vi "Convert SS2 Data Info to String.vi"(5 "File Path":path, 6 "Step Duration":dbl[unit] format="%#.3g", 7 "Laser Period":dbl[unit], 8 "error in (no error)":errorcluster, 9 "size":i64, 10 "# Frames":u32, 11 "Swiss SPAD 2 File Information":T1 {"DAQ Parameters"."# Gate Positions" format="%0.0f"; "DAQ Parameters"."Gate Offset" format="%0.0f"; "DAQ Parameters"."Bitness" format="%0.0f"; "DAQ Parameters"."# Gate Set" format="%0.0f"; "FPGA Parameters"."gs_psincdec 3" format="%0.0f"; "FPGA Parameters"."gs_psincdec 2" format="%0.0f"; "FPGA Parameters"."gs_psincdec_1" format="%0.0f"; "FPGA Parameters"."gs_no_shift_adj_3" format="%0.0f"; "FPGA Parameters"."gs_no_shift_adj_2" format="%0.0f"; "FPGA Parameters"."gs_psincdec_0" format="%0.0f"}) -> (0 "Error Out":errorcluster, 3 "Data Description":string)   [LabVIEW 2021, in "SwissSPAD.lvlib"]
uses:
  SwissSPAD.lvlib
  SS2 File Information.ctl
  SS2 FPGA Parameters.ctl
  SS2 DAQ Parameters.ctl
  SS2 Data Information.ctl
  SwissSPAD 8-bit Frames Read.ctl
  Variant/Variant.lvlib
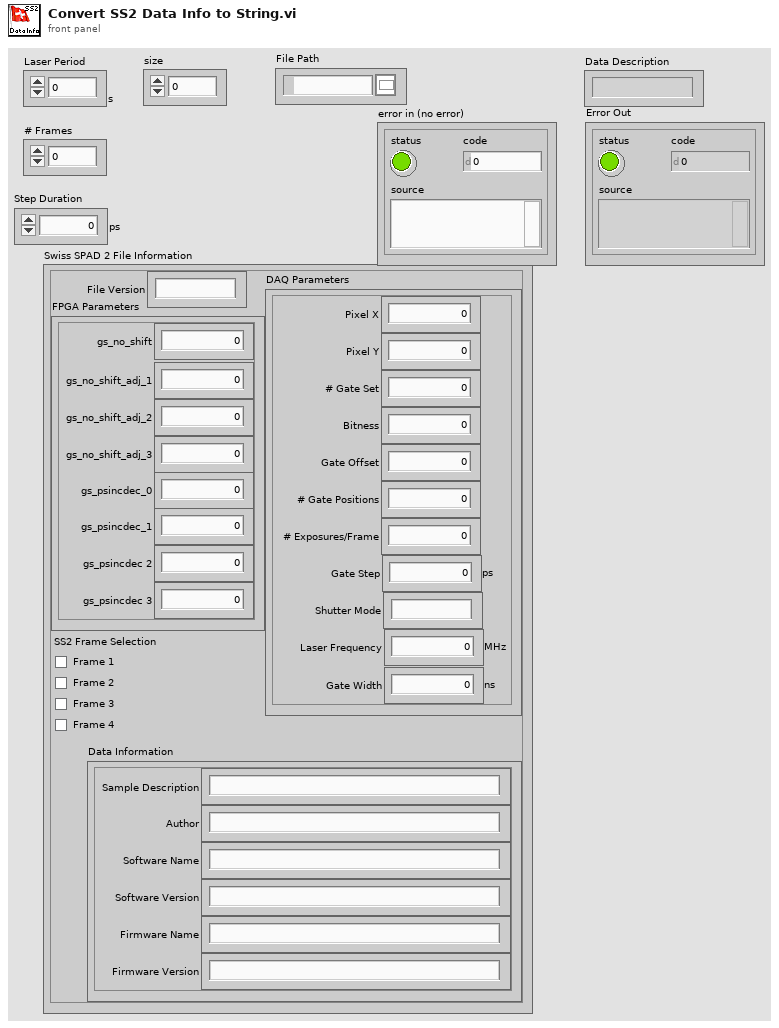
[diagram p1: front panel]
types:
  T1 = typedef "SwissSPAD.lvlib/SS2 File Information.ctl" = cluster{"File Version":string, "FPGA Parameters":T2, "DAQ Parameters":T3, "Data Information":T4, "SS2 Frame Selection":T5}
  T2 = typedef "SwissSPAD.lvlib/SS2 FPGA Parameters.ctl" = cluster{"gs_no_shift":i32, "gs_no_shift_adj_1":u32, "gs_no_shift_adj_2":u32, "gs_no_shift_adj_3":u32, "gs_psincdec_0":i32, "gs_psincdec_1":u32, "gs_psincdec 2":u32, "gs_psincdec 3":u32}
  T3 = typedef "SwissSPAD.lvlib/SS2 DAQ Parameters.ctl" = cluster{"Pixel X":i32, "Pixel Y":i32, "# Gate Set":i32, "Bitness":i32, "Gate Offset":i32, "# Gate Positions":i32, "# Exposures/Frame ":i32, "Gate Step":dbl[unit], "Shutter Mode":string, "Laser Frequency":dbl[unit], "Gate Width":dbl[unit]}
  T4 = typedef "SwissSPAD.lvlib/SS2 Data Information.ctl" = cluster{"Sample Description":string, "Author":string, "Software Name":string, "Software Version":string, "Firmware Name":string, "Firmware Version":string}
  T5 = typedef "SwissSPAD.lvlib/SwissSPAD 8-bit Frames Read.ctl" = cluster{"Frame 1":bool, "Frame 2":bool, "Frame 3":bool, "Frame 4":bool}
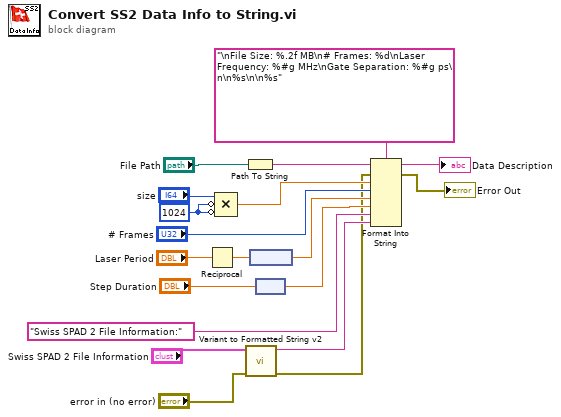
[diagram p0: block diagram]
diagram:
  w13 = i64 1024 ("y")
  n1 = Reciprocal(x="Laser Period") -> (1/x=w9:dbl[unit])
  n2 = Compound Arithmetic op=MULTIPLY("size", invert w13, invert w13) -> (w12:dbl)
  n3 = Path To String(path="File Path") -> (string=w16:string)
  n4 = call "Variant to Formatted String v2.vi"("error in (no error)"="error in (no error)", "Anything"="Swiss SPAD 2 File Information") -> ("error out"=w3:errorcluster, "String"=w4:string)  [unwired: 8 in]
  n5 = node(w9) -> (w8:dbl)
  n6 = node("Step Duration") -> (w6:dbl)
  n7 = Format Into String(format string="\nFile Size: %.2f MB\n# Frames: %d\nLaser Frequency: %#g MHz\nGate Separation: %#g ps\n\n%s\n\n%s", initial string=w16, error in=w3, w12, "# Frames", w8, w6, "Swiss SPAD 2 File Information:" ("Label"), w4) -> (resulting string=→"Data Description":string, error out=→"Error Out":errorcluster)
